vi "Get DataArray (String).vi"(8 "error in (no error)":errorcluster, 11 "DataGridView in":refnum<class "DataGridView.lvclass">) -> (0 "error out":errorcluster, 2 "Array":string[][](array[string]), 3 "DataGridView out":refnum<class "DataGridView.lvclass">)   [LabVIEW 2016, in "DataGrid.lvlib" / "DataGridView.lvclass"]
uses:
  <userlib>/LabVIEWdotNetDataGrid/source/DataGridView/DataGridView.lvclass
  <userlib>/LabVIEWdotNetDataGrid/source/DataGridView/DataGridView.lvclass/DataGridView.ctl
  <userlib>/LabVIEWdotNetDataGrid/source/DataTable/DataTable.lvclass
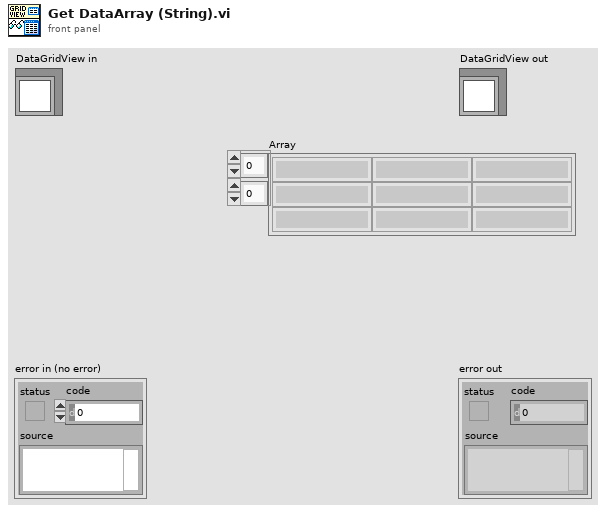
[diagram p1: front panel]
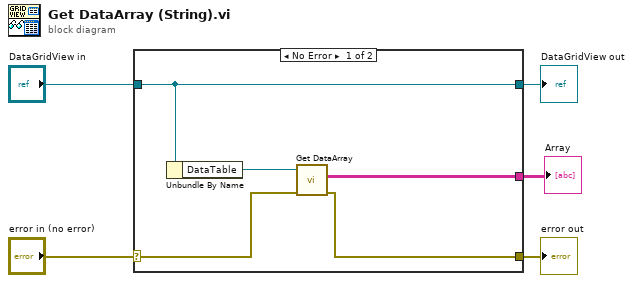
[diagram p0: block diagram]
diagram:
  n1 = case shown="No Error" "error in (no error)" {
    selector: "error in (no error)" -> [w8 w11]
    tunnel: [w7 w11] -> w4
    tunnel: [w10 w12] -> w2
    tunnel: "DataGridView in" -> [w10 w12]
    tunnel: [w6 _] -> w1
    frame No Error {
      n2 = Unbundle By Name(w10) -> ("DataTable"=w9:refnum<class "DataTable.lvclass">)
      n3 = call-poly <userlib>:"Get DataArray.vi"("error in (no error)"=w8, "DataTable in"=w9) -> ("error out"=w7:errorcluster, "Array"=w6:string[][])  [unwired: 7 in, 1 out]
    }
    frame Error {
    }
  }
  "error out" <- w4
  "DataGridView out" <- w2
  "Array" <- w1
